vi "SVD backsub.vi"(2 "A":dbl[](array[numeric]), 3 "V":T1, 4 "1/S":T1, 5 "U^T":T1) -> (0 "error out":errorcluster, 1 "solution":dbl[](array[numeric]) format="%.2f")   [LabVIEW 2020, in "NI_Gmath.lvlib"]
uses:
  <vilib>/gmath/NI_Gmath.lvlib
  <vilib>/Analysis/Matrix/Datatypes/RealMatrix.ctl
  <vilib>/Analysis/baseanly.llb/A x Vector.vi
  <vilib>/Analysis/NI_AALBase.lvlib
  <vilib>/Analysis/Matrix/NI_Matrix.lvlib
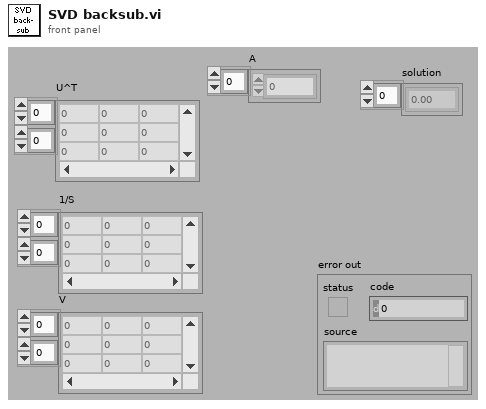
[diagram p1: front panel]
types:
  T1 = typedef "NI_Matrix.lvlib/RealMatrix.ctl" = dbl[][]
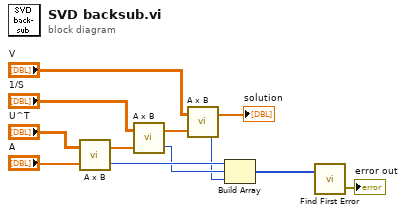
[diagram p0: block diagram]
diagram:
  n1 = call-poly <vilib>:"A x B.vi"("Vector"="A", "A"="U^T") -> ("error"=w5:i32, "A x Vector"=w10:dbl[])
  n2 = call-poly <vilib>:"A x B.vi"("Vector"=w10, "A"="1/S") -> ("error"=w4:i32, "A x Vector"=w8:dbl[])
  n3 = call-poly <vilib>:"A x B.vi"("Vector"=w8, "A"="V") -> ("error"=w3:i32, "A x Vector"=→"solution":dbl[])
  n4 = Build Array(w5, w4, w3) -> (w2:i32[])
  n5 = call <vilib>:"Find First Error.vi"("error codes"=w2) -> ("error out"=→"error out":errorcluster)  [unwired: 3 in, 1 out]
